vi "_Remote Run Dual.vi"(4 "error in":errorcluster) -> (0 "error out":errorcluster)   [LabVIEW 2015]
uses:
  Type/_RT Command.ctl
  Type/_RT Parameter.ctl
  Type/_RT Active Ch.ctl
  Type/_RT Expt.ctl
  Type/_Run Mode.ctl
  Type/_RT Mass Range.ctl
  Type/_RT Res Type.ctl
  Type/_Ramp Parameter.ctl
  Configuration/_Global Configuration.vi
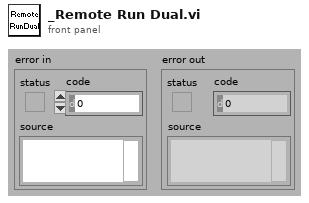
[diagram p1: front panel]
types:
  T1 = typedef "_Ramp Parameter.ctl" = cluster{"Name":string, "Channel":u8, "Offset":dbl, "Slope":dbl, "Count 1":dbl, "Count 2":dbl, "Time 1":dbl, "Time 2":dbl, "Scans":i32, "Step Size":dbl}
  T2 = typedef "_RT Expt.ctl" = cluster{"StartT(mS)":i32, "#Cycles":i32, "Scan Type":T3, "PauseT(uS)":i32, "Polarity":u8, "DelayT(mS)":i32, "Active Ch":T4[], "Mass Range":T5[]}
  T3 = typedef "_Run Mode.ctl" = enum16{"MRM (Q1/Q2)", "Q1 Scan", "Q1 SRM", "Q2 Scan", "Q2 SRM", "Product Scan", "Precursor Scan", "Neutral Loss", "Neutral Gain"}
  T4 = typedef "_RT Active Ch.ctl" = cluster{"Start":i32, "Step":i32, "ChID":i32}
  T5 = typedef "_RT Mass Range.ctl" = cluster{"Steps":i32, "Dwell(uS)":i32, "Resolution Type":T6, "Ramping Ch":T4[]}
  T6 = typedef "_RT Res Type.ctl" = u16
  T7 = typedef "_RT Parameter.ctl" = cluster{"RunMode":i32, "Initial Ch":T4[], "Sync":u8, "Expt":T2[], "EqTime(mS)":i32}
  T8 = typedef "_RT Command.ctl" = enum16{"xml Start Run", "xml Start Actual Run", "xml Stop Run", "xml Runtime Update", "xml Get Status", "xml Get Table", "xml Set Table", "xml Get Configuration", "xml System Status", "xml Set LC Input Logic", "xml Get Data", "xml Get Info", "Start", "StartActualRun", "Stop", "Runtime Update", "Get Data", "Get Info", "Get Status", "Get Param", "Get Config", "Get Table", "Read ADC", "Set Oscillator", "Update Config", "Update Table", "Set All Pol", "Set Pol and DC", "Set Max Mass", "Toggle RP", "Toggle EL", "Set PIC", "Initialize Turbo", "Send Turbo Comm", "Close Turbo", "P1", "P2", "P3", "Send Serial", "Set LC Out", "Get LC In", "Read VAC", "Test Table", "Toggle Power", "Get Startup", "Set Startup", "Get ADC Table", "Set ADC Table", "Get Brief Status", "Get Detail Status", "Auxiliary Update", "Set CC Logics", "Set CC Input Logics", "Ignore Error", "invalid"}
  T9 = typedef "_RT Instrument 2.ctl" = cluster{"Table":T10[], "Instrument":string[]}
  T10 = typedef "_RT Configuration 2.ctl" = cluster{"Name":string, "Ch#":u8, "Min":dbl, "Max":dbl, "Def+":dbl, "Def-":dbl, "Offset":dbl, "Slope":dbl, "Type":u8, "Description":string, "SettleT":dbl}
  T11 = typedef "_Lens Property.ctl" = cluster{"Scan Type":u8, "Scans":i32, "Time 1":dbl, "Time 2":dbl, "Value 1":dbl, "Value 2":dbl, "Step Size":dbl}
  T12 = typedef "_Mass Range Property.ctl" = cluster{"Start":dbl, "Stop":dbl, "Step Size":dbl, "Steps":i32, "Dwell":dbl, "Parameters":T13[], "Res":T6}
  T13 = typedef "_Mass Range Parameters.ctl" = cluster{"Name":string, "Ch#":u8, "StartV":dbl, "StopV":dbl, "StepV":dbl, "Index":u8}
  T14 = cluster{"Lenses":T11[], "Mass Ranges":T12[], "Acquire":bool, "MCA":bool, "Q1DC EN":bool, "Q1 POL":bool, "Q3 POL":bool, "Q1 RF  EN":bool, "Averaging":bool, "Log Scale":bool, "CPS":bool, "Unit":bool, "Data Path":path, "Run Mode":T3, "Fixed Mass (amu)":dbl, "Q3DC EN":bool, "Q3 RF  EN":bool, "Negative":bool}
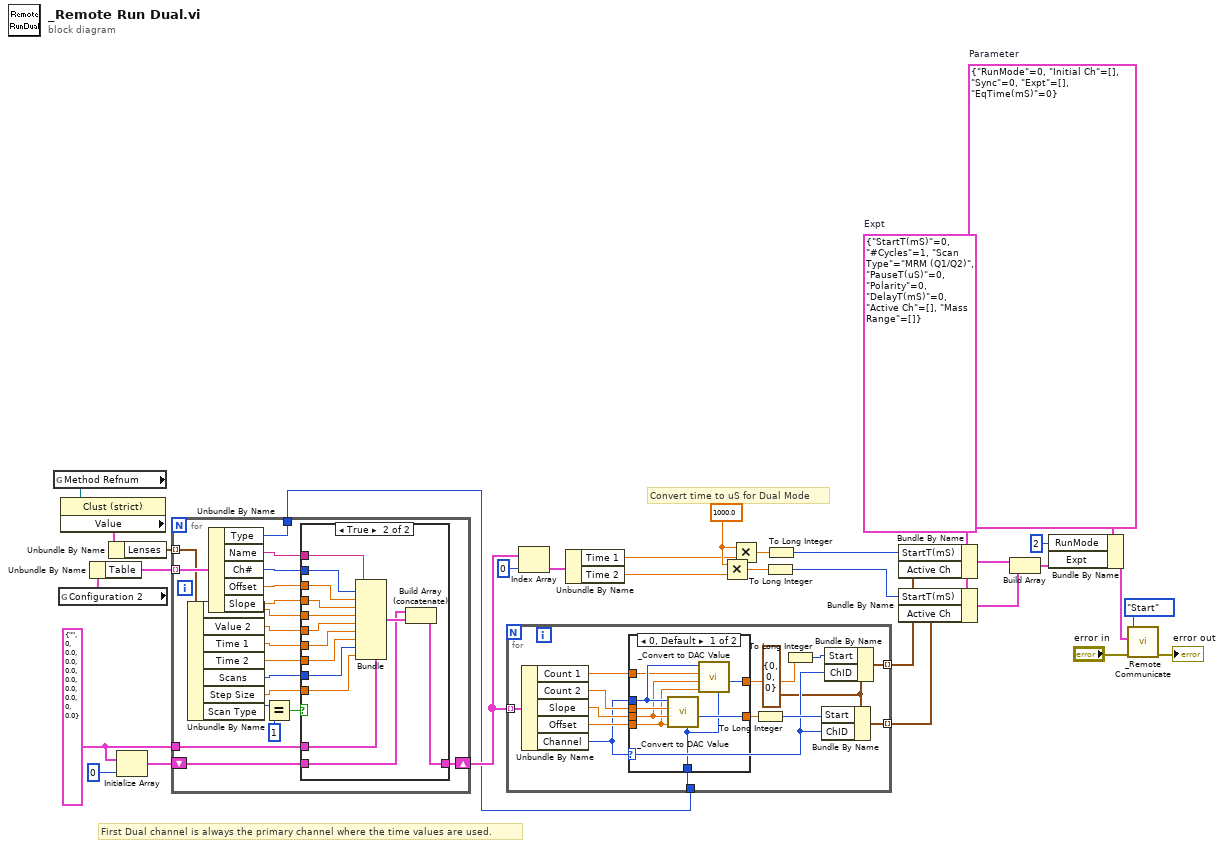
[diagram p0: block diagram]
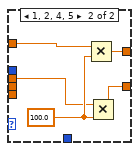
[diagram p2: hidden frame]
diagram:
  w10 = T1 {"Name"="", "Channel"=0, "Offset"=0.0, "Slope"=0.0, "Count 1"=0.0, "Count 2"=0.0, "Time 1"=0.0, "Time 2"=0.0, "Scans"=0, "Step Size"=0.0} ("Ramp Parameter")
  w17 = 1000.0 ("x")
  w23 = T2 {"StartT(mS)"=0, "#Cycles"=1, "Scan Type"=enum."MRM (Q1/Q2)", "PauseT(uS)"=0, "Polarity"=0, "DelayT(mS)"=0, "Active Ch"=[], "Mass Range"=[]}  # Expt
  w25 = T7 {"RunMode"=0, "Initial Ch"=[], "Sync"=0, "Expt"=[], "EqTime(mS)"=0}  # Parameter
  # "First Dual channel is always the primary channel where the time values are used."
  # "Convert time to uS for Dual Mode"
  n1 = global read "_Global Configuration.vi" "Method Refnum"() -> (w14:refnum<vi>)
  n2 = global read "_Global Configuration.vi" "Configuration 2"() -> (w12:T9)
  n3 = property class="Clust (strict)"(reference=w14) -> ("Value"=w15:T14)  [unwired: 1 in, 2 out]
  n4 = Unbundle By Name(w12) -> ("Table"=w13:T10[])
  n5 = Unbundle By Name(w15) -> ("Lenses"=w16:T11[])
  n6 = Initialize Array(w10, 0 ("dimension size")) -> (w9:T1[])
  n7 = for {
    shift-right: [w44] -> w8
    shift-left: w9 -> [w45]
    tunnel: w10 -> [w43]
    tunnel: w13 -> [w42] mode=indexing
    tunnel: w16 -> [w41] mode=indexing
    tunnel: [w32] -> w1
    n8 = Unbundle By Name(w41) -> ("Value 1"=w40:dbl, "Value 2"=w39:dbl, "Time 1"=w38:dbl, "Time 2"=w37:dbl, "Scans"=w36:i32, "Step Size"=w35:dbl, "Scan Type"=w34:u8)
    n9 = Unbundle By Name(w42) -> ("Type"=w32:u8, "Name"=w49:string, "Ch#"=w48:u8, "Offset"=w47:dbl, "Slope"=w46:dbl)
    n10 = Equal?(x=w34, y=u8 1) -> (x = y?=w50:bool)
    n11 = case shown="True" w50 {
      tunnel: w40 -> [_ w65]
      tunnel: w49 -> [_ w64]
      tunnel: w48 -> [_ w63]
      tunnel: w47 -> [_ w62]
      tunnel: w46 -> [_ w61]
      tunnel: w39 -> [_ w60]
      tunnel: w38 -> [_ w53]
      tunnel: w37 -> [_ w52]
      tunnel: w36 -> [_ w59]
      tunnel: w35 -> [_ w58]
      tunnel: w45 -> [w51 w56]
      tunnel: [w51 w54] -> w44
      tunnel: w43 -> [_ w55]
      frame False {
      }
      frame True {
        n12 = Bundle(cluster=w55, "Name"=w64, "Channel"=w63, "Offset"=w62, "Slope"=w61, "Count 1"=w65, "Count 2"=w60, "Time 1"=w53, "Time 2"=w52, "Scans"=w59, "Step Size"=w58) -> (w57:T1)
        n13 = Build Array (concatenate)(w56, w57) -> (w54:T1[])
      }
    }
  }
  n14 = for {
    tunnel: w8 -> [w79] mode=indexing
    tunnel: [w72] -> w5 mode=indexing
    tunnel: [w68] -> w4 mode=indexing
    tunnel: w1 -> [w66]
    w67 = T4 {"Start"=0, "Step"=0, "ChID"=0} ("Active Channel")
    n15 = Unbundle By Name(w79) -> ("Count 1"=w73:dbl, "Count 2"=w77:dbl, "Slope"=w76:dbl, "Offset"=w75:dbl, "Channel"=w69:u8)
    n16 = case shown="0, Default" w69 {
      tunnel: [w86 w88] -> w78
      tunnel: w69 -> [w85 _]
      tunnel: w77 -> [w87 w90]
      tunnel: w76 -> [w83 _]
      tunnel: w75 -> [w82 _]
      tunnel: w73 -> [w84 w91]
      tunnel: [w81 w89] -> w70
      tunnel: w66 -> [w80 _]
      frame 0, Default {
        n17 = call "_Convert to DAC Value.vi"("Type"=w80, "Offset"=w82, "Slop"=w83, "Number"=w87, "Channel"=w85) -> ("DAC Value"=w86:i32)  [unwired: 1 in, 5 out]
        n18 = call "_Convert to DAC Value.vi"("Type"=w80, "Offset"=w82, "Slop"=w83, "Number"=w84, "Channel"=w85) -> ("DAC Value"=w81:i32)  [unwired: 1 in, 5 out]
      }
      frame 1, 2, 4, 5 {
        w92 = 100.0 ("y")
        n19 = Multiply(x=w91, y=w92) -> (x*y=w89:dbl)
        n20 = Multiply(x=w90, y=w92) -> (x*y=w88:dbl)
      }
    }
    n21 = To Long Integer(number=w78) -> (32bit integer=w74:i32)
    n22 = To Long Integer(number=w70) -> (32bit integer=w71:i32)
    n23 = Bundle By Name(cluster=w67, "Start"=w74, "ChID"=w69) -> (w72:T4)
    n24 = Bundle By Name(cluster=w67, "Start"=w71, "ChID"=w69) -> (w68:T4)
  }
  n25 = Index Array(array=w8, index=0) -> (element=w6:T1)
  n26 = Unbundle By Name(w6) -> ("Time 1"=w3:dbl, "Time 2"=w2:dbl)
  n27 = Multiply(x=w17, y=w2) -> (x*y=w19:dbl)
  n28 = Multiply(x=w17, y=w3) -> (x*y=w18:dbl)
  n29 = To Long Integer(number=w19) -> (32bit integer=w20:i32)
  n30 = To Long Integer(number=w18) -> (32bit integer=w21:i32)
  n31 = Bundle By Name(cluster=w23, "StartT(mS)"=w21, "Active Ch"=w4) -> (w27:T2)
  n32 = Bundle By Name(cluster=w23, "StartT(mS)"=w20, "Active Ch"=w5) -> (w22:T2)
  n33 = Build Array(w27, w22) -> (w28:T2[])
  n34 = Bundle By Name(cluster=w25, "RunMode"=2, "Expt"=w28) -> (w24:T7)
  n35 = call "_Remote Communicate.vi"("error in (no error)"="error in", "Parameter"=w24, "Command"=_RT_Command."Start") -> ("error out"=→"error out":errorcluster)  [unwired: 3 in, 3 out]
